vi "lsb_offset.vi"() -> ()   [LabVIEW 2018]
uses:
  <vilib>/rvi/eio/common/nirviEmuTemplateMethod_errors.vi
  <vilib>/rvi/eio/common/nirviEmuTemplatePropertyGet_noerrors.vi
  <vilib>/eio/EIONode/EIONode.xnode
  <vilib>/eio/EIOPropertyNode/EIOPropertyNode.xnode
  <vilib>/rvi/eio/common/nirviEmuTemplatePropertyGet_errors.vi
  <vilib>/rvi/eio/common/nirviEmuTemplatePropertySet_errors.vi
  <vilib>/rvi/eio/common/nirviEmuTemplatePropertySet_noerrors.vi
panel:
  out "Cluster0":cluster{"LSB Weight":u32, "Offset":i32}
  out "Cluster1":cluster{"LSB Weight":u32, "Offset":i32}
  out "Cluster2":cluster{"LSB Weight":u32, "Offset":i32}
  out "Cluster3":cluster{"LSB Weight":u32, "Offset":i32}
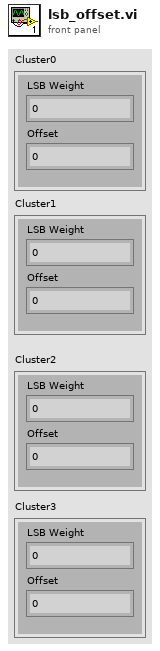
[diagram p1: front panel]
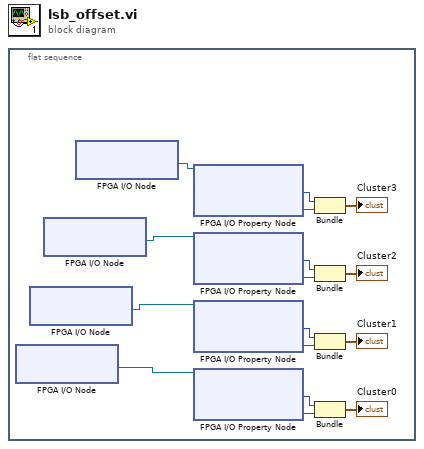
[diagram p0: block diagram]
diagram:
  n1 = flat-sequence {
    frame #0 {
      n2 = xnode "FPGA I/O Node"() -> ("FPGA I/O Out"=w1:refnum<k21>)  [unwired: 1 in, 1 out]
      n3 = xnode "FPGA I/O Node"() -> ("FPGA I/O Out"=w2:refnum<k21>)  [unwired: 1 in, 1 out]
      n4 = xnode "FPGA I/O Node"() -> ("FPGA I/O Out"=w3:refnum<k21>)  [unwired: 1 in, 1 out]
      n5 = xnode "FPGA I/O Node"() -> ("FPGA I/O Out"=w4:refnum<k21>)  [unwired: 1 in, 1 out]
      n6 = xnode "FPGA I/O Property Node"("FPGA I/O In"=w4) -> ("LSB Weight"=w14:u32, "Offset"=w15:i32)  [unwired: 1 out]
      n7 = xnode "FPGA I/O Property Node"("FPGA I/O In"=w3) -> ("LSB Weight"=w11:u32, "Offset"=w12:i32)  [unwired: 1 out]
      n8 = xnode "FPGA I/O Property Node"("FPGA I/O In"=w2) -> ("LSB Weight"=w8:u32, "Offset"=w9:i32)  [unwired: 1 out]
      n9 = xnode "FPGA I/O Property Node"("FPGA I/O In"=w1) -> ("LSB Weight"=w5:u32, "Offset"=w6:i32)  [unwired: 1 out]
      n10 = Bundle("LSB Weight"=w14, "Offset"=w15) -> (→"Cluster3":cluster{"LSB Weight":u32, "Offset":i32})  [unwired: 1 in]
      n11 = Bundle("LSB Weight"=w11, "Offset"=w12) -> (→"Cluster2":cluster{"LSB Weight":u32, "Offset":i32})  [unwired: 1 in]
      n12 = Bundle("LSB Weight"=w8, "Offset"=w9) -> (→"Cluster1":cluster{"LSB Weight":u32, "Offset":i32})  [unwired: 1 in]
      n13 = Bundle("LSB Weight"=w5, "Offset"=w6) -> (→"Cluster0":cluster{"LSB Weight":u32, "Offset":i32})  [unwired: 1 in]
    }
  }
